vi "Get laser power.vi"(11 "VISA resource name":refnum<visa-resource-name>) -> (2 "Laser Power":dbl(slide) min=0.0 max=120.0 step=1.0 scale=0.0..100.0 scale format="%.1f", 3 "VISA resource name out":refnum<visa-resource-name>)   [LabVIEW 2017]
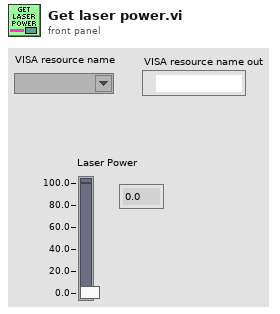
[diagram p1: front panel]
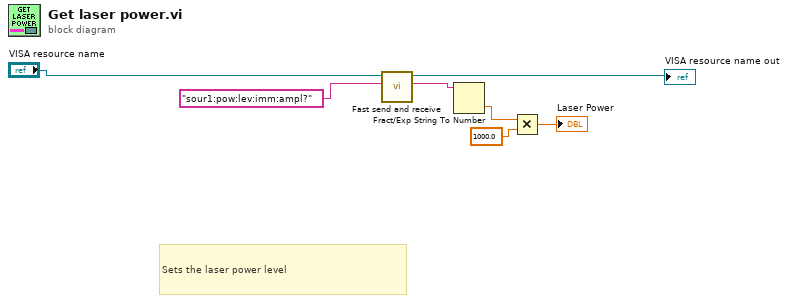
[diagram p0: block diagram]
diagram:
  # "Sets the laser power level"
  n1 = call "Fast send and receive.vi"("write to laser"="sour1:pow:lev:imm:ampl?", "VISA resource name"="VISA resource name") -> ("read from laser"=w2:string, "VISA resource name out"=→"VISA resource name out":refnum<visa-resource-name>)  [unwired: 8 in]
  n2 = Fract/Exp String To Number(string=w2) -> (number=w4:dbl)  [unwired: 3 in, 1 out]
  n3 = Multiply(x=w4, y=1000.0) -> (x*y=→"Laser Power":dbl)
